vi "CreateJsonComment.vi"(10 "Variant":variant) -> (2 "String":string)   [LabVIEW 2018, in "Matlab.lvclass"]
uses:
  Matlab.lvclass
  <vilib>/addons/_JKI.lib/Serialization/JSON/JKI JSON Serialization.lvlib
  <vilib>/Utility/Data Type/NI_Data Type.lvlib
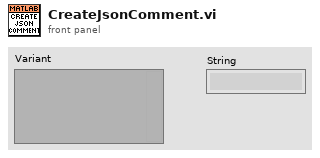
[diagram p1: front panel]
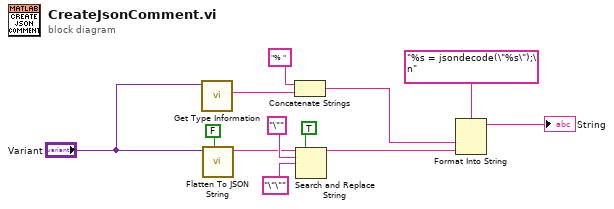
[diagram p0: block diagram]
diagram:
  n1 = call <vilib>:"Get Type Information.vi"("Variant"="Variant") -> ("Name"=w4:string)  [unwired: 6 in, 4 out]
  n2 = call <vilib>:"Flatten To JSON String.vi"("Multiline (T)"=FALSE, "Variant"="Variant") -> ("JSON String"=w5:string)  [unwired: 8 in, 1 out]
  n3 = Concatenate Strings("% " ("string"), w4) -> (w1:string)
  n4 = Search and Replace String(replace all?=TRUE ("replace all? (F)"), input string=w5, search string="\"", replace string="\"\"" ("search string")) -> (result string=w2:string)  [unwired: 4 in, 3 out]
  n5 = Format Into String(format string="%s = jsondecode(\"%s\");\n", w1, w2) -> (resulting string=→"String":string)  [unwired: 2 in, 1 out]
